vi "TakeSampleImage.vi"(6 "SampleName":string, 7 "MotorController in":refnum<class "MotorController.lvclass">, 8 "Error In":errorcluster, 9 "Exposure":u16, 10 "Angles":i64[](array[numeric]), 11 "TLCamera reference in":refnum<k24>) -> (0 "Error Out":errorcluster, 2 "Image Array":u16[][](array[numeric]), 3 "TLCamera reference out":refnum<k24>, 5 "MotorController out":refnum<class "MotorController.lvclass">)   [LabVIEW 2019]
uses:
  MotorController.lvclass
  C:/Users/jleeman/git_repos/CAxis_Machine/C-Axis LabView Controller/Library_X64/Thorlabs.TSI.TLCameraInterfaces.dll
  Library_X64/Thorlabs.TSI.TLCameraInterfaces.dll
panel:
  out "path":path
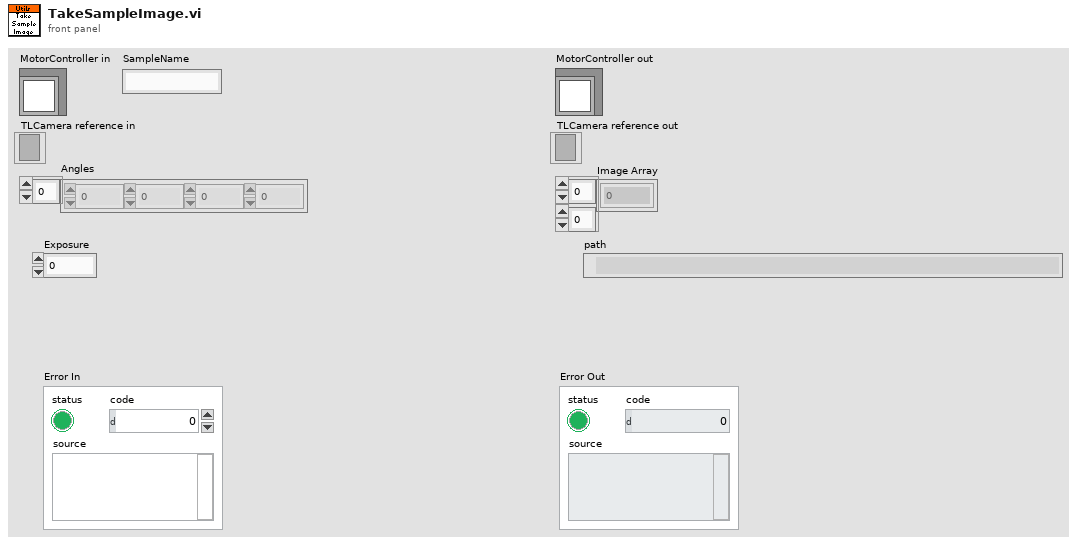
[diagram p1: front panel]
types:
  T1 = typedef "IMAQ Image.ctl" = refnum<image>
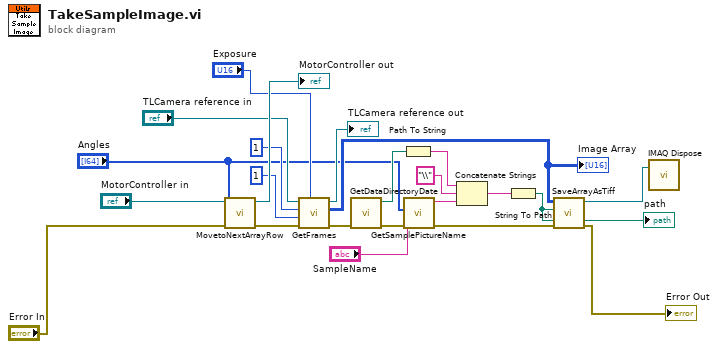
[diagram p0: block diagram]
diagram:
  n1 = call "MovetoNextArrayRow.vi"("Error In"="Error In", "Positions"="Angles", "MotorController in"="MotorController in") -> ("Error Out"=w12:errorcluster, "MotorController out"=→"MotorController out":refnum<class "MotorController.lvclass">)  [unwired: 7 in]
  n2 = call "GetFrames.vi"("ExposureTime_us"="Exposure", "Error In"=w12, "FramesPerTrigger"=u32 1, "Gain"=u32 1, "TLCamera reference in"="TLCamera reference in") -> ("Error Out"=w11:errorcluster, "Array"=w7:u16[][], "TLCamera reference out"=→"TLCamera reference out":refnum<k24>)  [unwired: 4 in]
  "Image Array" <- w7
  n3 = call "GetDataDirectoryDate.vi"("Error In"=w11) -> ("Error Out"=w10:errorcluster, "path"=w23:path)  [unwired: 9 in]
  n4 = Path To String(path=w23) -> (string=w22:string)
  n5 = call "GetSamplePictureName.vi"("Error In"=w10, "Array"="Angles", "SampleName"="SampleName") -> ("Error Out"=w6:errorcluster, "filename"=w9:string)  [unwired: 7 in]
  n6 = Concatenate Strings(w22, "\\" ("string"), w9) -> (w20:string)
  n7 = String To Path(string=w20) -> (path=w8:path)
  "path" <- w8
  n8 = call "SaveArrayAsTiff.vi"("Error In"=w6, "File Path"=w8, "Array"=w7) -> ("Error Out"=→"Error Out":errorcluster, "Image Out"=w1:T1)  [unwired: 7 in]
  n9 = call "IMAQ Dispose"("Image"=w1) -> ()  [unwired: 5 in, 1 out]
